vi "DSF.Engine.Runtime.Framework.Get CPU Info.vi"(8 "error in (no error)":errorcluster, 11 "Framework Runtime in":refnum<class "DSF.Engine.Runtime.Framework.lvclass">) -> (0 "error out":errorcluster, 2 "CPU Info":T1 {"caches"."cache entry size" format="%d bytes"; "caches"."total cache size" format="%d bytes"}, 3 "Framework Runtime out":refnum<class "DSF.Engine.Runtime.Framework.lvclass">)   [LabVIEW 2016, in "DSF.Engine.lvlib" / "DSF.Engine.Runtime.Framework.lvclass"]
uses:
  DSF.Engine.Runtime.Framework.lvclass
  DSF.Engine.Typedefs.CPU Info.ctl
  DSF.Engine.lvlib
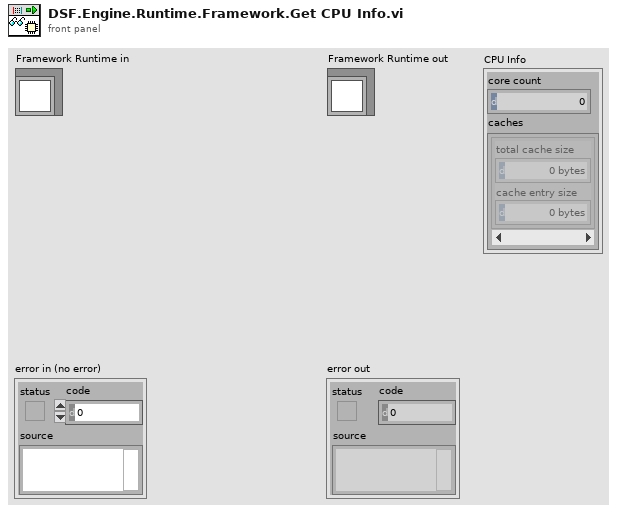
[diagram p1: front panel]
types:
  T1 = typedef "DSF.Engine.lvlib/DSF.Engine.Typedefs.CPU Info.ctl" = cluster{"core count":i32, "caches":cluster{"total cache size":i32, "cache entry size":i32}[]}
  T2 = cluster{"total cache size":i32, "cache entry size":i32}
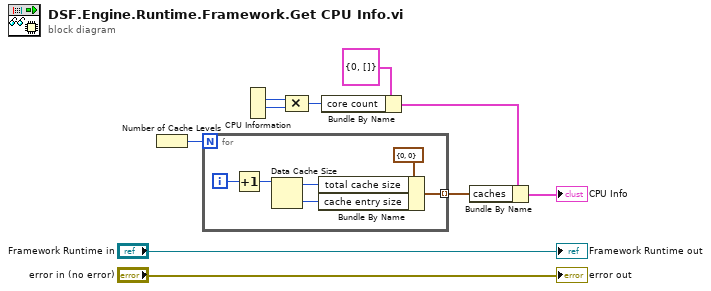
[diagram p0: block diagram]
diagram:
  n1 = Number of Cache Levels() -> (w7:i32)
  n2 = for {
    N: w7 -> [_]
    tunnel: [w13] -> w6 mode=indexing
    i -> [w12]
    n3 = Increment(x=w12) -> (x+1=w11:i32)
    n4 = Data Cache Size(0:w11) -> (4:w14:i32, 7:w15:i32)
    n5 = Bundle By Name(cluster=T2 {"total cache size"=0, "cache entry size"=0} ("caches"), "total cache size"=w14, "cache entry size"=w15) -> (w13:T2)
  }
  n6 = CPU Information() -> (5:w2:i32, 6:w3:i32)  [unwired: 2 out]
  n7 = Compound Arithmetic op=MULTIPLY(w2, w3) -> (w1:i32)
  n8 = Bundle By Name(cluster=T1 {"core count"=0, "caches"=[]} ("CPU Info"), "core count"=w1) -> (w5:T1)
  n9 = Bundle By Name(cluster=w5, "caches"=w6) -> (→"CPU Info":T1)
  "error out" <- "error in (no error)"
  "Framework Runtime out" <- "Framework Runtime in"
